vi "Flattening JSON Object to Array of JSON Paths.vi"() -> ()   [LabVIEW 2019]
doc: "Example of taking a nested JSON Object structure and flalttening it to an array of JSONpaths and corresponding JSON Values."
uses:
  vi.lib/JDP Science/JSONtext/JSONtext.lvlib
panel:
  in  "Include $Paths to Objects":bool
  out "<JSON>Reassembled":string
  out "<JSON>Items":string[](array[string])
  out "$Paths":string[](array[string])
  in  "JSON Object":string="{\"widget\": {\n    \"debug\": \"on\",\n    \"example.dot.in.name\":true,\n    \"window\": {\n        \"title\": \"Sample Konfabulator Widget\",\n        \"name\": \"main_window\",\n        \"width\": 500,\n        \"height\": 500\n    },\n    \"image\": { \n        \"src\": \"Images/Sun.png\",\n        \"name\": \"sun1\",\n        \"hOffset\": 250,\n        \"vOffset\": 250,\n        \"alignment\": \"center\"\n    },\n    \"text\": {\n        \"data\": \"Click Here\",\n        \"size\": 36,\n        \"style\": \"bold\",\n        \"name\": \"text1\",\n        \"hOffset\": 250,\n        \"vOffset\": 100,\n        \"alignment\": \"center\",\n        \"onMouseUp\": \"sun1.opacity = (sun1.opacity / 100) * 90;\"\n    }\n}} "
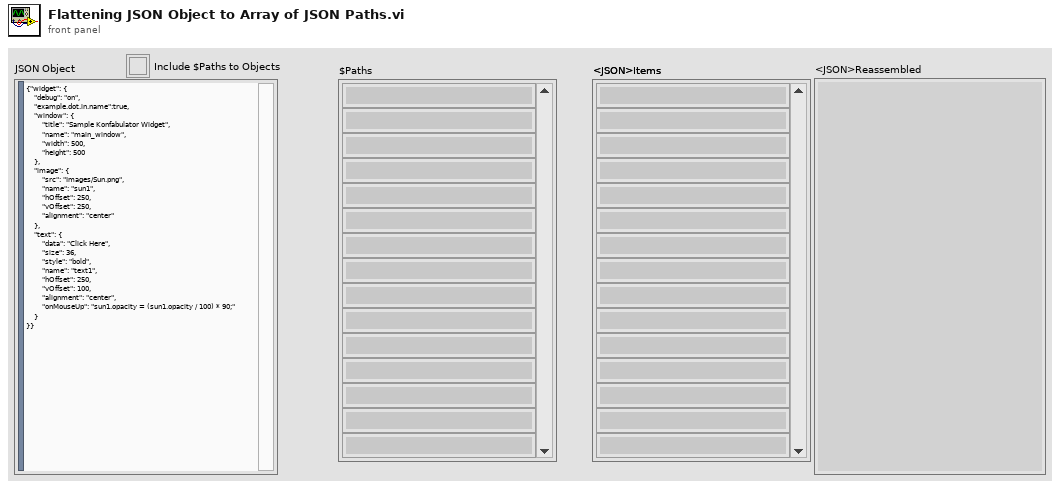
[diagram p1: front panel]
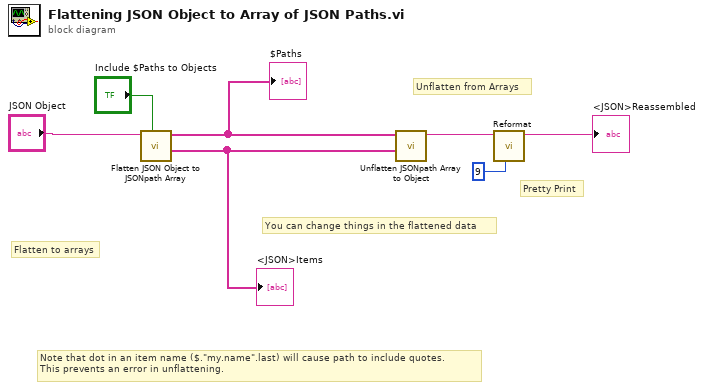
[diagram p0: block diagram]
diagram:
  # "Note that dot in an item name ($.\"my.name\".last) will cause path to include quotes.\nThis prevents an error in unflattening."
  # "Unflatten from Arrays"
  # "Flatten to arrays"
  # "You can change things in the flattened data"
  # "Pretty Print"
  n1 = call "Flatten JSON Object to JSONpath Array.vi"("Include $Paths to Objects"="Include $Paths to Objects", "JSON"="JSON Object") -> ("<JSON>"=w5:string[], "$Paths"=w6:string[])  [unwired: 7 in, 1 out]
  "$Paths" <- w6
  "<JSON>Items" <- w5
  n2 = call "Unflatten JSONpath Array to Object.vi"("JSON Items"=w5, "$Paths"=w6) -> ("<JSON>"=w4:string)  [unwired: 8 in, 1 out]
  n3 = call "Reformat.vi"("Pretty Print Levels"=9, "JSON"=w4) -> ("<JSON>"=→"<JSON>Reassembled":string)  [unwired: 6 in, 3 out]
